vi "FlatToRichnixnet_grpc_FrameBufferResponse.vi"(5 "OutputClusterType":T1, 11 "InputCluster":T2) -> (3 "OutputCluster":T1)   [LabVIEW 2024, in "grpc-xnet_client.lvlib"]
uses:
  grpc-xnet_client.lvlib
  nixnet_grpc_FrameBufferResponse_frame/nixnet_grpc_FrameBufferResponse_frame.lvclass
  nixnet_grpc_FrameBufferResponse_frame/nixnet_grpc_FrameBufferResponse_frame.lvclass/nixnet_grpc_FrameBufferResponse_frame.ctl
  nixnet_grpc_FrameBufferResponse.ctl
  nixnet_grpc_EnetFlags.ctl
  nixnet_grpc_EnetFrameType.ctl
  nixnet_grpc_EnetFrameResponse_Flat.ctl
  nixnet_grpc_FrameFlags.ctl
  nixnet_grpc_FrameType.ctl
  nixnet_grpc_FrameResponse_Flat.ctl
  nixnet_grpc_FrameBufferResponse_Flat.ctl
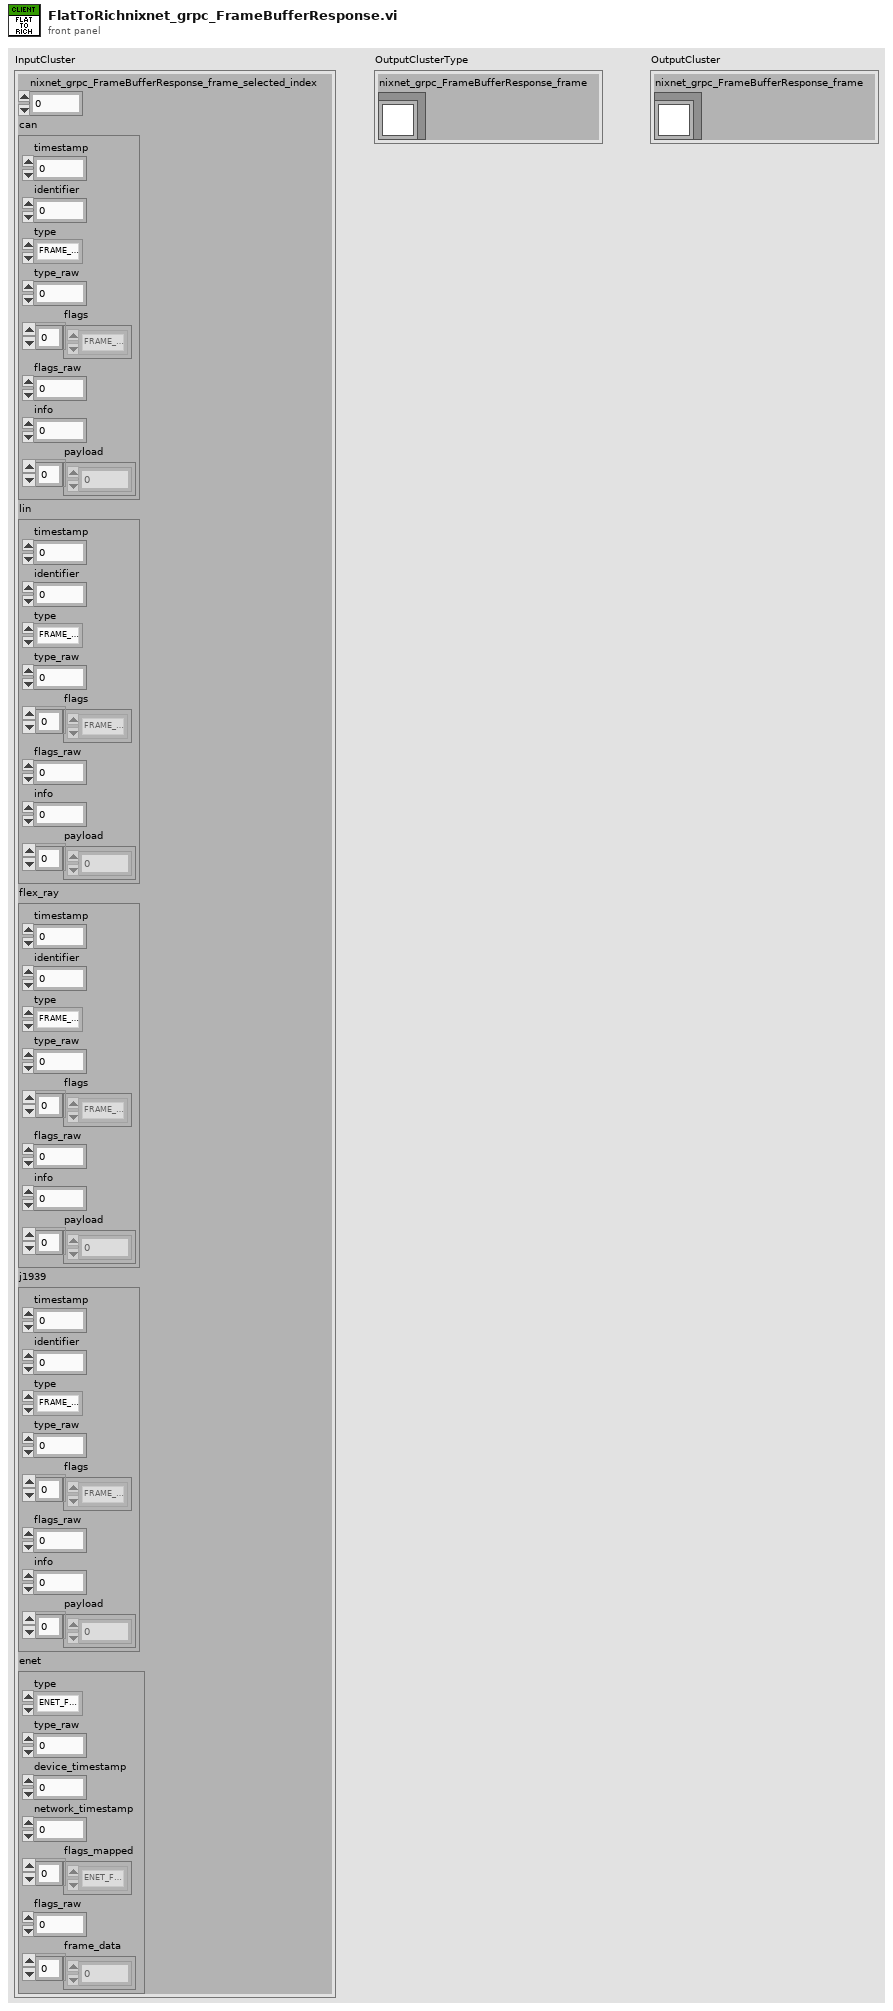
[diagram p1: front panel]
types:
  T1 = typedef "grpc-xnet_client.lvlib/nixnet_grpc_FrameBufferResponse.ctl" = cluster{"nixnet_grpc_FrameBufferResponse_frame":refnum<class "nixnet_grpc_FrameBufferResponse_frame.lvclass">}
  T2 = typedef "grpc-xnet_client.lvlib/nixnet_grpc_FrameBufferResponse_Flat.ctl" = cluster{"nixnet_grpc_FrameBufferResponse_frame_selected_index":i32, "can":T3, "lin":T3, "flex_ray":T3, "j1939":T3, "enet":T6}
  T3 = typedef "grpc-xnet_client.lvlib/nixnet_grpc_FrameResponse_Flat.ctl" = cluster{"timestamp":u64, "identifier":u32, "type":T4, "type_raw":u32, "flags":T5[], "flags_raw":u32, "info":u32, "payload":u8[]}
  T4 = typedef "grpc-xnet_client.lvlib/nixnet_grpc_FrameType.ctl" = enum32{"FRAME_TYPE_CAN_DATA", "FRAME_TYPE_CAN_REMOTE", "FRAME_TYPE_CAN_BUS_ERROR", "FRAME_TYPE_CAN20_DATA", "FRAME_TYPE_CANFD_DATA", "FRAME_TYPE_CANFDBRS_DATA", "FRAME_TYPE_FLEX_RAY_DATA", "FRAME_TYPE_FLEX_RAY_NULL", "FRAME_TYPE_FLEX_RAY_SYMBOL", "FRAME_TYPE_LIN_DATA", "FRAME_TYPE_LIN_BUS_ERROR", "FRAME_TYPE_LIN_NO_RESPONSE", "FRAME_TYPE_J1939_DATA", "FRAME_TYPE_SPECIAL_DELAY", "FRAME_TYPE_SPECIAL_LOG_TRIGGER", "FRAME_TYPE_SPECIAL_START_TRIGGER"}
  T5 = typedef "grpc-xnet_client.lvlib/nixnet_grpc_FrameFlags.ctl" = enum32{"FRAME_FLAGS_UNSPECIFIED", "FRAME_FLAGS_FLEX_RAY_STARTUP", "FRAME_FLAGS_FLEX_RAY_SYNC", "FRAME_FLAGS_FLEX_RAY_PREAMBLE", "FRAME_FLAGS_FLEX_RAY_CH_A", "FRAME_FLAGS_FLEX_RAY_CH_B", "FRAME_FLAGS_LIN_EVENT_SLOT", "FRAME_FLAGS_TRANSMIT_ECHO"}
  T6 = typedef "grpc-xnet_client.lvlib/nixnet_grpc_EnetFrameResponse_Flat.ctl" = cluster{"type":T7, "type_raw":u32, "device_timestamp":u64, "network_timestamp":u64, "flags_mapped":T8[], "flags_raw":u32, "frame_data":u8[]}
  T7 = typedef "grpc-xnet_client.lvlib/nixnet_grpc_EnetFrameType.ctl" = enum32{"ENET_FRAME_TYPE_DATA", "ENET_FRAME_TYPE_DELAY", "ENET_FRAME_TYPE_FUTURE_TIME_WAIT"}
  T8 = typedef "grpc-xnet_client.lvlib/nixnet_grpc_EnetFlags.ctl" = enum32{"ENET_FLAGS_UNSPECIFIED", "ENET_FLAGS_TRANSMIT", "ENET_FLAGS_RECEIVE", "ENET_FLAGS_NETWORK_SYNCED", "ENET_FLAGS_ERROR"}
  T9 = typedef "grpc-xnet_client.lvlib/nixnet_grpc_FrameResponse.ctl" = cluster{"timestamp":u64, "identifier":u32, "type":T4, "type_raw":u32, "flags":T5[], "flags_raw":u32, "info":u32, "payload":u8[]}
  T10 = typedef "grpc-xnet_client.lvlib/nixnet_grpc_EnetFrameResponse.ctl" = cluster{"type":T7, "type_raw":u32, "device_timestamp":u64, "network_timestamp":u64, "flags_mapped":T8[], "flags_raw":u32, "frame_data":u8[]}
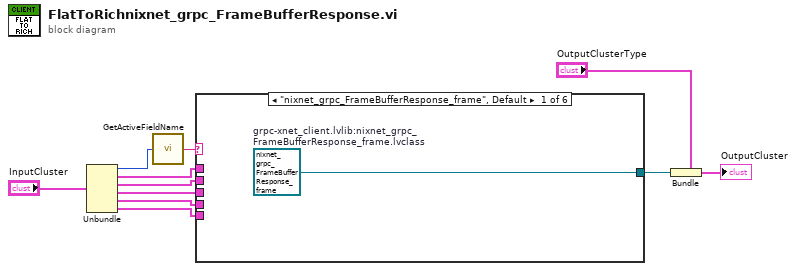
[diagram p0: block diagram]
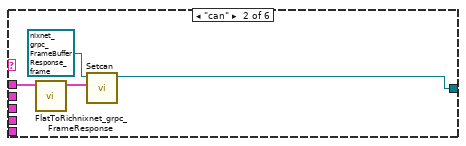
[diagram p2: hidden frame]
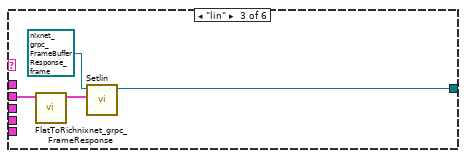
[diagram p3: hidden frame]
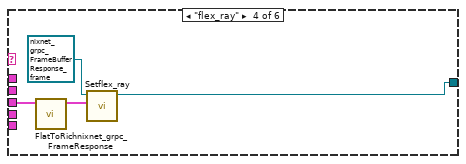
[diagram p4: hidden frame]
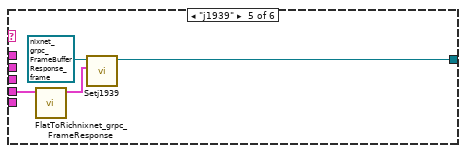
[diagram p5: hidden frame]
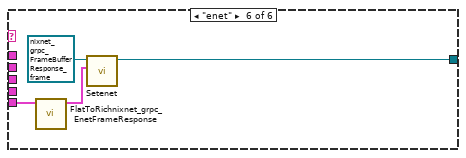
[diagram p6: hidden frame]
diagram:
  n1 = Unbundle "Unbundle"("InputCluster") -> ("nixnet_grpc_FrameBufferResponse_frame_selected_index"=w8:i32, "can"=w5:T3, "lin"=w4:T3, "flex_ray"=w3:T3, "j1939"=w2:T3, "enet"=w1:T6)
  n2 = call "GetActiveFieldName.vi"("protobuf index"=w8) -> ("oneof field name"=w7:string)
  n3 = case "nixnet_grpc_FrameBufferResponse_frame" shown="\"nixnet_grpc_FrameBufferResponse_frame\", Default" w7 {
    tunnel: [w12 w14 w18 w22 w26 w30] -> w6
    tunnel: w5 -> [_ w16 _ _ _ _]
    tunnel: w4 -> [_ _ w20 _ _ _]
    tunnel: w3 -> [_ _ _ w24 _ _]
    tunnel: w2 -> [_ _ _ _ w28 _]
    tunnel: w1 -> [_ _ _ _ _ w32]
    frame "nixnet_grpc_FrameBufferResponse_frame", Default {
      w12 = refnum<class "nixnet_grpc_FrameBufferResponse_frame.lvclass"> refnum  # grpc-xnet_client.lvlib:nixnet_grpc_FrameBufferResponse_frame.lvclass
    }
    frame "can" {
      n4 = call "FlatToRichnixnet_grpc_FrameResponse.vi"("InputCluster"=w16) -> ("OutputCluster"=w15:T9)  [unwired: 10 in]
      n5 = call "Setcan.vi"("Set_Val"=w15, "OneOfTemplate in"=refnum<class "nixnet_grpc_FrameBufferResponse_frame.lvclass"> refnum) -> ("OneOfTemplate out"=w14:refnum<class "nixnet_grpc_FrameBufferResponse_frame.lvclass">)  [unwired: 8 in, 1 out]
    }
    frame "lin" {
      n6 = call "FlatToRichnixnet_grpc_FrameResponse.vi"("InputCluster"=w20) -> ("OutputCluster"=w19:T9)  [unwired: 10 in]
      n7 = call "Setlin.vi"("Set_Val"=w19, "OneOfTemplate in"=refnum<class "nixnet_grpc_FrameBufferResponse_frame.lvclass"> refnum) -> ("OneOfTemplate out"=w18:refnum<class "nixnet_grpc_FrameBufferResponse_frame.lvclass">)  [unwired: 8 in, 1 out]
    }
    frame "flex_ray" {
      n8 = call "FlatToRichnixnet_grpc_FrameResponse.vi"("InputCluster"=w24) -> ("OutputCluster"=w23:T9)  [unwired: 10 in]
      n9 = call "Setflex_ray.vi"("Set_Val"=w23, "OneOfTemplate in"=refnum<class "nixnet_grpc_FrameBufferResponse_frame.lvclass"> refnum) -> ("OneOfTemplate out"=w22:refnum<class "nixnet_grpc_FrameBufferResponse_frame.lvclass">)  [unwired: 8 in, 1 out]
    }
    frame "j1939" {
      n10 = call "FlatToRichnixnet_grpc_FrameResponse.vi"("InputCluster"=w28) -> ("OutputCluster"=w27:T9)  [unwired: 10 in]
      n11 = call "Setj1939.vi"("Set_Val"=w27, "OneOfTemplate in"=refnum<class "nixnet_grpc_FrameBufferResponse_frame.lvclass"> refnum) -> ("OneOfTemplate out"=w26:refnum<class "nixnet_grpc_FrameBufferResponse_frame.lvclass">)  [unwired: 8 in, 1 out]
    }
    frame "enet" {
      n12 = call "FlatToRichnixnet_grpc_EnetFrameResponse.vi"("InputCluster"=w32) -> ("OutputCluster"=w31:T10)  [unwired: 10 in]
      n13 = call "Setenet.vi"("Set_Val"=w31, "OneOfTemplate in"=refnum<class "nixnet_grpc_FrameBufferResponse_frame.lvclass"> refnum) -> ("OneOfTemplate out"=w30:refnum<class "nixnet_grpc_FrameBufferResponse_frame.lvclass">)  [unwired: 8 in, 1 out]
    }
  }
  n14 = Bundle "Bundle"(cluster="OutputClusterType", "nixnet_grpc_FrameBufferResponse_frame"=w6) -> (→"OutputCluster":T1)
